vi "new Input Type Filter.vi"(10 "Input Type":T1(ring)) -> (2 "input type filter out":refnum<class "Filter.lvclass">)   [LabVIEW 2016, in "FPGA Resource Manager System Defintion.lvlib" / "Input Type Filter.lvclass"]
uses:
  Input Type Filter.lvclass
  Filter Parent/Filter.lvclass
  C:/github/VeriStand-FPGA-Resource-Manager/Source/Filters/Filter Parent/Filter.lvclass
  Input Type Filter.lvclass/Input Type Filter.ctl
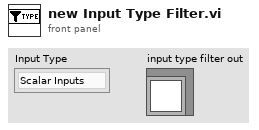
[diagram p1: front panel]
types:
  T1 = enum16{"Scalar Inputs", "Scalar Outputs", "Waveform Inputs", "Waveform Outputs"}
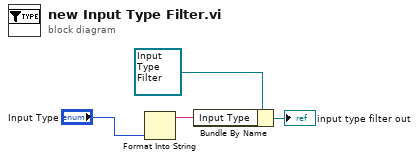
[diagram p0: block diagram]
diagram:
  n1 = Format Into String("Input Type") -> (resulting string=w1:string)  [unwired: 3 in, 1 out]
  n2 = Bundle By Name(cluster=refnum<class "Input Type Filter.lvclass"> refnum ("Input Type Filter in"), "Input Type"=w1) -> (→"input type filter out":refnum<class "Input Type Filter.lvclass">)
